vi "UI_Launcher.vi"(0 "reference in":refnum<class "GUI.lvclass">, 5 "error in (no error)":errorcluster) -> (14 "reference out":refnum<class "GUI.lvclass">, 19 "error out":errorcluster)   [LabVIEW 2019, in "GUI.lvclass"]
uses:
  GUI.lvclass
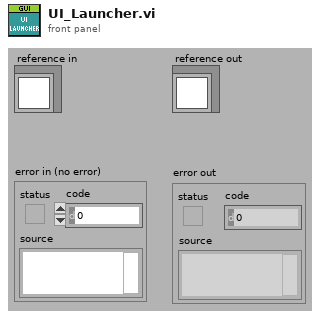
[diagram p1: front panel]
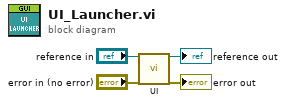
[diagram p0: block diagram]
diagram:
  n1 = call-dynamic "UI.vi"("reference in"="reference in", "error in (no error)"="error in (no error)") -> ("reference out"=→"reference out":refnum<class "GUI.lvclass">, "error out"=→"error out":errorcluster)  [unwired: 16 in]
